vi "step1.vi"(1 "NT":u32, 2 "C1":bool, 3 "NC1":u32, 6 "T":u32, 12 "N step":u32) -> (13 "N step out":u32, 14 "T NT":u32[](array[numeric]), 15 "C NC":cluster{"C":bool, "NC":u32}[](array[cluster]))   [LabVIEW 2019, in "Userlib.lvlib"]
uses:
  Userlib.lvlib
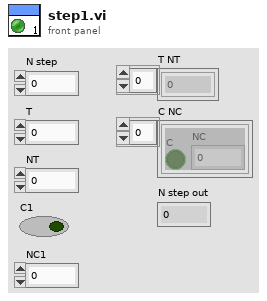
[diagram p1: front panel]
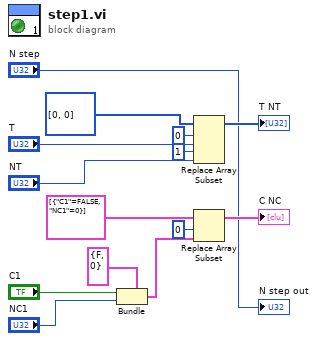
[diagram p0: block diagram]
diagram:
  n1 = Bundle(cluster=cluster{"C1":bool, "NC1":u32} {"C1"=FALSE, "NC1"=0}, "C1"="C1", "NC1"="NC1") -> (w3:cluster{"C1":bool, "NC1":u32})
  n2 = Replace Array Subset(array=u32[] [0, 0] ("appended array"), new element #1="T", index #1=0 ("index"), new element #2="NT", index #2=1 ("index")) -> (→"T NT":u32[])
  n3 = Replace Array Subset(array=cluster{"C1":bool, "NC1":u32}[] [{"C1"=FALSE, "NC1"=0}] ("appended array"), new element=w3, index=0) -> (→"C NC":cluster{"C1":bool, "NC1":u32}[])
  "N step out" <- "N step"
